vi "RT Cal procedure.vi"(7 "Top level fpga ref":refnum<k20>, 10 "FPGA out refs":refnum<k20>[](array[refnum]), 11 "FPGA in refs":refnum<k20>[](array[refnum])) -> (2 "FPGA out refs out":refnum<k20>[](array[refnum]), 3 "FPGA in refs out":refnum<k20>[](array[refnum]), 5 "Top level fpga ref out":refnum<k20>)   [LabVIEW 2014, in "UEGO Sim Engine.lvlib"]
uses:
  <vilib>/NI/LVFPGA Adv Session Resources/OpenByNameSubVI.vi
  <vilib>/Analysis/baseanly.llb/Mean (DBL).vi
  Shared/Constants.vi
  <vilib>/rvi/interface/common/dynamic/niFpgaEscapeDelimiterAndNull.vi
  <vilib>/Utility/error.llb/Error Cluster From Error Code.vi
  <vilib>/rvi/errors/niLvFpgaAdjustHostInterfaceError.vi
  <vilib>/NI/LVFPGA Adv Session Resources/OpenByName.xnode
  <vilib>/rvi/interface/nirviReadWriteControl/nirviReadWriteControl.xnode
  UEGO Sim Engine.lvlib
  Shared/UEGO Sim Shared.lvlib
  <vilib>/NI/LVFPGA Adv Session Resources/LVFPGAAdvSessionResources.lvlib
  NiFpgaLv.dll
  <vilib>/rvi/interface/Simulation/niFpgaSimulationCallBeginRW.vi
  <vilib>/Analysis/NI_AALBase.lvlib
panel:
  out "error out":errorcluster
  in  "Error In":errorcluster
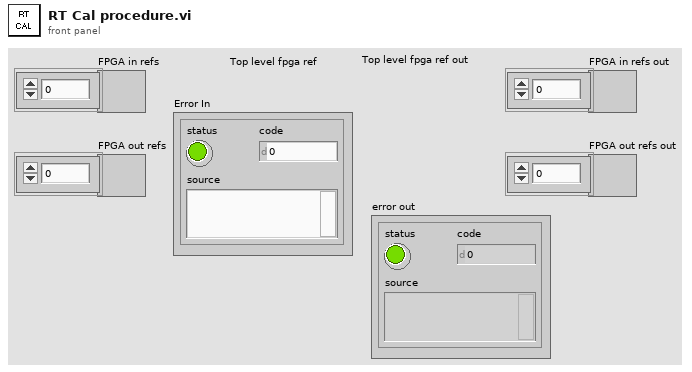
[diagram p1: front panel]
types:
  T1 = cluster{"Name":string, "Depth":u32, "Write? (Deprecated:Use Implementation)":bool, "Physical Channel":u32, "Base Address":u32, "Data Width":u32, "Data Type":enum32{"Boolean", "I8", "I16", "I32", "I64", "U8", "U16", "U32", "U64", "FXP", "CustomControl", "SGL"}, "FXP Properties":variant, "Write Window Address":u32, "Implementation":enum16{"niFpgaTargetToHost", "niFpgaHostToTarget", "niFpgaPeerToPeerWriter", "niFpgaPeerToPeerReader", "niCoreTargetToHost", "niCoreHostToTarget"}, "Control Set":u32}[]
  T2 = cluster{"Name":string, "type":variant, "indicator?":bool}[]
  T3 = cluster{"Sensor Model":enum16{"Narrow Band", "Bosch 4.2", "Bosch 4.9"}, "lambda":fxp<+,12,3>, "cal":bool, "negate":bool, "PWM threshold":i16, "PWM timeout":u32}
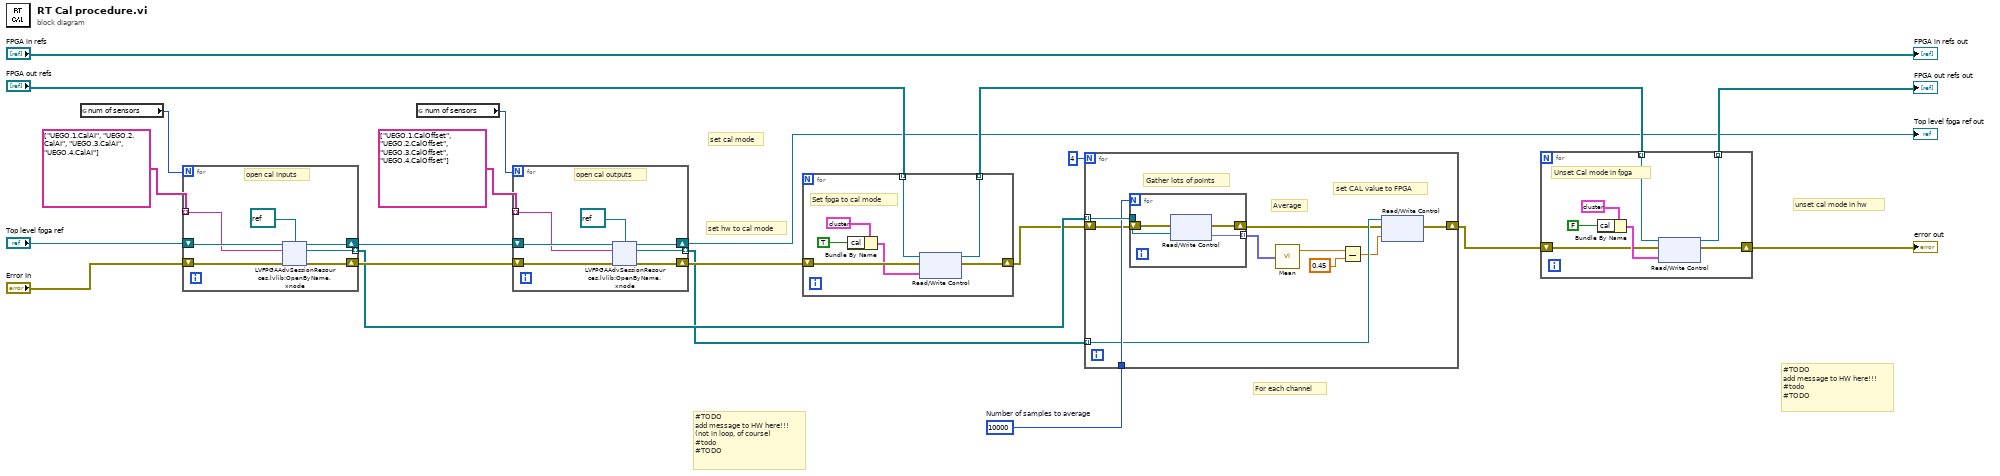
[diagram p0: block diagram]
diagram:
  w4 = 10000  # Number of samples to average
  # "For each channel"
  # "set hw to cal mode"
  # "#TODO\nadd message to HW here!!!\n#todo\n#TODO"
  # "unset cal mode in hw"
  # "#TODO\nadd message to HW here!!!\n(not in loop, of course)\n#todo\n#TODO"
  # "set cal mode"
  n1 = global read "Constants.vi" "num of sensors"() -> (w20:i32)
  n2 = for {
    N: w20 -> [_]
    tunnel: string[] ["UEGO.1.CalAI", "UEGO.2.CalAI", "UEGO.3.CalAI", "UEGO.4.CalAI"] -> [w26] mode=indexing
    tunnel: [w24] -> w5 mode=indexing
    shift-right: [w23] -> w14
    shift-left: "Error In" -> [w27]
    shift-right: [w22] -> w15
    shift-left: "Top level fpga ref" -> [w28]
    # "open cal inputs"
    n3 = xnode "LVFPGAAdvSessionResources.lvlib:OpenByName.xnode"("FPGA VI Reference in"=w28, "Resource name in"=w26, "Single resource reference type in"=refnum<k20> refnum, "Error in"=w27) -> ("Single resource reference out"=w24:refnum<k20>, "Error out"=w23:errorcluster, "FPGA VI Reference out"=w22:refnum<k20>)
  }
  n4 = global read "Constants.vi" "num of sensors"() -> (w19:i32)
  n5 = for {
    N: w19 -> [_]
    tunnel: string[] ["UEGO.1.CalOffset", "UEGO.2.CalOffset", "UEGO.3.CalOffset", "UEGO.4.CalOffset"] -> [w46] mode=indexing
    tunnel: [w44] -> w3 mode=indexing
    shift-right: [w43] -> w12
    shift-left: w14 -> [w47]
    shift-right: [w42] -> w8
    shift-left: w15 -> [w48]
    # "open cal outputs"
    n6 = xnode "LVFPGAAdvSessionResources.lvlib:OpenByName.xnode"("FPGA VI Reference in"=w48, "Resource name in"=w46, "Single resource reference type in"=refnum<k20> refnum, "Error in"=w47) -> ("Single resource reference out"=w44:refnum<k20>, "Error out"=w43:errorcluster, "FPGA VI Reference out"=w42:refnum<k20>)
  }
  "Top level fpga ref out" <- w8
  n7 = for {
    tunnel: "FPGA out refs" -> [w68] mode=indexing
    tunnel: [w64] -> w11 mode=indexing
    shift-right: [w62] -> w2
    shift-left: w12 -> [w67]
    # "Set fpga to cal mode"
    n8 = Bundle By Name(cluster=T3 {"Sensor Model"=enum."Narrow Band", "lambda"=0.0, "cal"=FALSE, "negate"=FALSE, "PWM threshold"=0, "PWM timeout"=0} ("Value"), "cal"=TRUE) -> (w63:T3)
    n9 = xnode "Read/Write Control"("FPGA VI Reference In"=w68, "error in"=w67, "Value"=w63) -> ("FPGA VI Reference Out"=w64:refnum<k20>, "error out"=w62:errorcluster)
  }
  n10 = for {
    N: 4 -> [_]
    tunnel: w5 -> [w78] mode=indexing
    tunnel: w4 -> [w77]
    tunnel: w3 -> [w73] mode=indexing
    shift-right: [w69] -> w1
    shift-left: w2 -> [w71]
    # "set CAL value to FPGA"
    # "Average"
    # "Gather lots of points"
    n11 = for {
      N: w77 -> [_]
      tunnel: w78 -> [w82]
      tunnel: [w81] -> w76 mode=indexing
      shift-right: [w79] -> w70
      shift-left: w71 -> [w80]
      n12 = xnode "Read/Write Control"("FPGA VI Reference In"=w82, "error in"=w80) -> ("error out"=w79:errorcluster, "Value"=w81:fxp<+/-,28,6>)  [unwired: 1 out]
    }
    n13 = call-poly <vilib>:"Mean.vi"("X"=w76) -> ("mean"=w75:dbl)  [unwired: 1 out]
    n14 = Subtract(x=w75, y=0.45) -> (x-y=w72:dbl)
    n15 = xnode "Read/Write Control"("FPGA VI Reference In"=w73, "error in"=w70, "Value"=w72) -> ("error out"=w69:errorcluster)  [unwired: 1 out]
  }
  n16 = for {
    tunnel: w11 -> [w89] mode=indexing
    tunnel: [w86] -> w10 mode=indexing
    shift-right: [w84] -> w7
    shift-left: w1 -> [w83]
    # "Unset Cal mode in fpga"
    n17 = Bundle By Name(cluster=T3 {"Sensor Model"=enum."Narrow Band", "lambda"=0.0, "cal"=FALSE, "negate"=FALSE, "PWM threshold"=0, "PWM timeout"=0} ("Value"), "cal"=FALSE) -> (w85:T3)
    n18 = xnode "Read/Write Control"("FPGA VI Reference In"=w89, "error in"=w83, "Value"=w85) -> ("FPGA VI Reference Out"=w86:refnum<k20>, "error out"=w84:errorcluster)
  }
  "FPGA out refs out" <- w10
  "error out" <- w7
  "FPGA in refs out" <- "FPGA in refs"
